vi "BRig_RT__Case_Exp__endTrial_checkFreeReward.vi"(6 "input_dataBlock":u16[][](array[numeric]), 8 "input_dataExp":u16[](array[numeric]), 9 "input_dataTrial":u16[][](array[numeric]), 10 "input_dataCurrent":u16[](array[numeric])) -> (3 "output_state":T1, 5 "output_endBlock":bool)   [LabVIEW 2014]
uses:
  myRIO_BRig_RT__Case_Exp_stateList.ctl
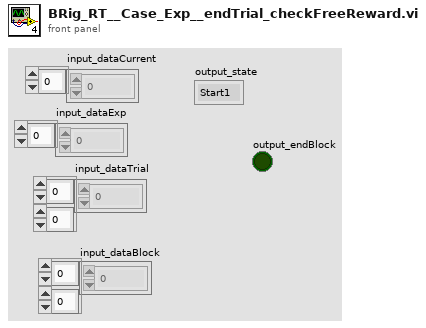
[diagram p1: front panel]
types:
  T1 = typedef "myRIO_BRig_RT__Case_Exp_stateList.ctl" = enum16{"Start1", "Start2", "Start3", "saveSettings1", "saveSettings2", "saveSettings3", "saveSettings4", "saveSettings_LC_ENL_l1", "saveSettings_LC_ENL_l2", "saveSettings_LC_Cue_l1", "saveSettings_LC_Cue_l2", "saveSettings6_LC_l1_Other", "SaveSettings6_LC_l2_Other", "setSettings_Audio", "setSettings_Laser", "initBlock_pre", "initBlock", "initBlock2", "initBlock_post", "initTrial_pre", "initTrial", "initTrial2", "initTrial3", "initTrial4", "initTrial_LC_ENL1", "initTrial_LC_Cue1", "initTrial_LC_Cue1_2", "initTrial_LC_Sel", "initTrial_post", "ENL1_pre", "ENL1", "ENL1_post", "ENL1Penalty_pre", "ENL1Penalty", "ENL2_pre", "ENL2", "ENL2Penalty_pre", "ENL2Penalty", "Cue1_pre", "Cue1", "Cue1_post", "Cue1Penalty_pre", "Cue1Penalty", "Cue2_pre", "Cue2", "Cue2Penalty_pre", "Cue2Penalty", "Selection_pre", "Selection", "Select_post", "SelectReward_pre", "SelectReward", "SelectRewardPost_pre", "SelectRewardPost", "SelectWrong_pre", "SelectWrong", "SelectWrong_post", "SelectTimeout_pre", "SelectTimeout", "SelectTimeout_post", "endTrial_pre", "endTrial1", "endTrial2", "endTrial3", "endTrial_post", "endBlock_pre", "endBlock", "endBlock_post", "endExp", "commConnect", "commUpload_pre", "commUpload_dataBlock", "commUpload_dataCurrent", "commUpload_dataExp", "commUpload_dataLC", "commUpload_dataTrial", "commUpload_post", "saveData_pre", "saveData_dataBlock", "saveData_dataCurrent", "saveData_dataExp", "saveData_dataLC", "saveData_dataTrial", "saveData_post", "empty_endBlock1", "empty_endBlock2", "empty_endTrial1", "empty_endTrial2", "empty_endTrial3", "empty_endTrial4", "empty_endTrial5", "dummyState", "dummyState_endBlock", "FreeReward_pre", "FreeReward", "FreeRewardPost_pre", "FreeRewardPost"}
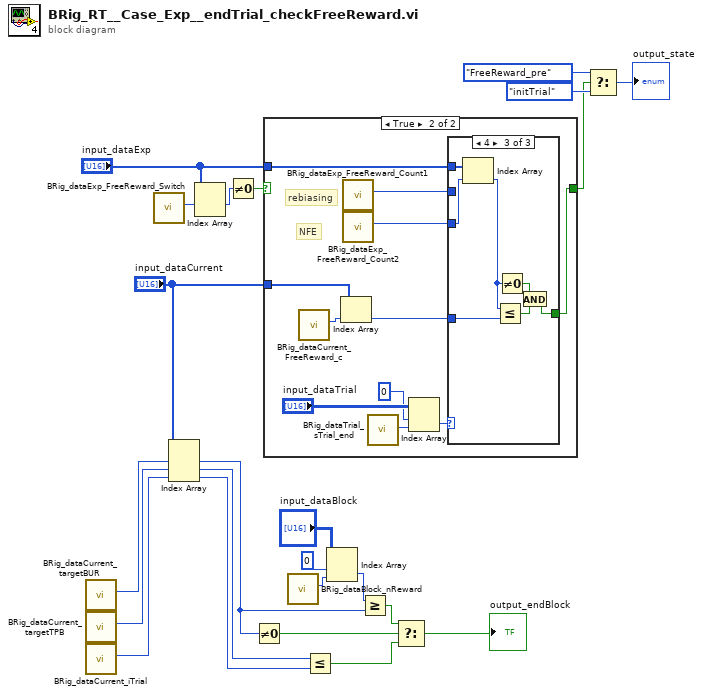
[diagram p0: block diagram]
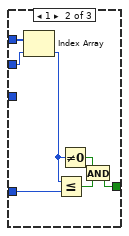
[diagram p4: hidden frame]
diagram:
  n1 = call "BRig_dataCurrent_targetBUR.vi"() -> ("output_targetBUR"=w3:i32)  [unwired: 11 in]
  n2 = call "BRig_dataCurrent_targetTPB.vi"() -> ("output_targetTPB"=w2:i32)  [unwired: 11 in]
  n3 = call "BRig_dataCurrent_iTrial.vi"() -> ("output_iTrial"=w4:i32)  [unwired: 11 in]
  n4 = call "BRig_dataExp_FreeReward_Switch.vi"() -> ("output_FreeReward_Switch"=w21:i32)  [unwired: 11 in]
  n5 = Index Array(array="input_dataCurrent", index #1=w3, index #2=w2, index #3=w4) -> (element #1=w12:u16, element #2=w5:u16, element #3=w6:u16)
  n6 = Index Array(array="input_dataExp", index #1=w21) -> (element #1=w20:u16)  [unwired: 1 in, 1 out]
  n7 = Not Equal To 0?(x=w20) -> (x != 0?=w19:bool)
  n8 = Not Equal To 0?(x=w12) -> (x != 0?=w7:bool)
  n9 = case shown="True" w19 {
    selector: w19 -> [w24 _]
    tunnel: "input_dataExp" -> [_ w31]
    tunnel: [w24 w27] -> w17
    tunnel: "input_dataCurrent" -> [_ w25]
    frame False {
    }
    frame True {
      # "NFE"
      # "rebiasing"
      n10 = call "BRig_dataCurrent_FreeReward_c.vi"() -> ("output_FreeReward_c"=w35:i32)  [unwired: 11 in]
      n11 = Index Array(array=w25, index=w35) -> (element=w28:u16)
      n12 = call "BRig_dataExp_FreeReward_Count1.vi"() -> ("output_FreeReward_Count"=w30:i32)  [unwired: 11 in]
      n13 = call "BRig_dataExp_FreeReward_Count2.vi"() -> ("output_FreeReward_Count"=w29:i32)  [unwired: 11 in]
      n14 = call "BRig_dataTrial_sTrial_end.vi"() -> ("output_sTrial_end"=w34:i32)  [unwired: 11 in]
      n15 = Index Array(array="input_dataTrial", index (row)=0, index (col)=w34) -> (element=w32:u16)
      n16 = case shown="4" w32 {
        tunnel: w31 -> [_ w42 w49]
        tunnel: w30 -> [_ w41 _]
        tunnel: w29 -> [_ _ w47]
        tunnel: w28 -> [_ w40 w48]
        tunnel: [_ w36 w43] -> w27
        frame 0, Default {
        }
        frame 1 {
          n17 = Index Array(array=w42, index=w41) -> (element=w39:u16)
          n18 = Less Or Equal?(x=w39, y=w40) -> (x <= y?=w38:bool)
          n19 = Not Equal To 0?(x=w39) -> (x != 0?=w37:bool)
          n20 = And(x=w37, y=w38) -> (x .and. y?=w36:bool)
        }
        frame 4 {
          n21 = Index Array(array=w49, index=w47) -> (element=w45:u16)
          n22 = Less Or Equal?(x=w45, y=w48) -> (x <= y?=w44:bool)
          n23 = Not Equal To 0?(x=w45) -> (x != 0?=w46:bool)
          n24 = And(x=w46, y=w44) -> (x .and. y?=w43:bool)
        }
      }
    }
  }
  n25 = call "BRig_dataBlock_nReward.vi"() -> ("output_nReward"=w10:i32)  [unwired: 11 in]
  n26 = Less Or Equal?(x=w5, y=w6) -> (x <= y?=w8:bool)
  n27 = Index Array(array="input_dataBlock", index (row)=0, index (col)=w10) -> (element=w11:u16)
  n28 = Greater Or Equal?(x=w11, y=w12) -> (x >= y?=w13:bool)
  n29 = Select(t=w13, s=w7, f=w8) -> (s? t:f=→"output_endBlock":bool)
  n30 = Select(t=myRIO_BRig_RT__Case_Exp_stateList."FreeReward_pre" ("Enum"), s=w17, f=myRIO_BRig_RT__Case_Exp_stateList."initTrial" ("Enum")) -> (s? t:f=→"output_state":T1)
